vi "Fix EtherCAT Error.vi"(8 "error in (no error)":errorcluster) -> (0 "error out":errorcluster)   [LabVIEW 2015, in "NI Synchronization Engine.lvlib"]
uses:
  NI Synchronization Engine.lvlib
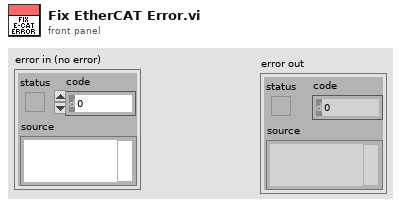
[diagram p1: front panel]
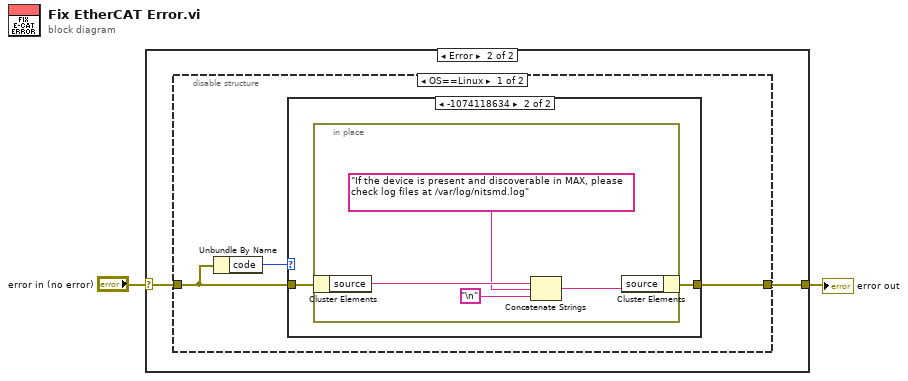
[diagram p0: block diagram]
diagram:
  n1 = case shown="Error" "error in (no error)" {
    selector: "error in (no error)" -> [w3 w5]
    tunnel: [w3 w4] -> w2
    frame No Error {
    }
    frame Error {
      n2 = disable-structure shown="OS==Linux" {
        disable-tunnel: w5 -> [w6 w16]
        disable-tunnel: [w7 w16] -> w4
        frame condition #0 (active) {
          n3 = Unbundle By Name(w6) -> ("code"=w8:i32)
          n4 = case shown="-1074118634" w8 {
            tunnel: [w9 w10] -> w7
            tunnel: w6 -> [w9 w11]
            frame Default {
            }
            frame -1074118634 {
              n5 = in-place {
                n6 = in-place-cluster #1(w11) -> ("source"=w14:string)
                n7 = Concatenate Strings(w14, "If the device is present and discoverable in MAX, please check log files at /var/log/nitsmd.log" ("string"), "\n") -> (w15:string)
                n8 = in-place-cluster #1("source"=w15) -> (w10:errorcluster)
              }
            }
          }
        }
        frame condition #1 {
        }
      }
    }
  }
  "error out" <- w2
